vi "itc ltc plots.vi"(4 "Plot: heater/gas":refnum<vi>, 5 "aggregate every # sec":dbl=1.0, 6 "Plot: temperature":refnum<vi>, 7 "plot length (min)":dbl=20.0, 8 "plot?":bool=TRUE, 10 "temperature indicator panel":T1={"LTC T"=0.0, "ITC T"=299.2, "ITC Set T"=295.0, "LTC T slope, K/min"=-0.0, "heater i-average, V"=-0.0, "heater slope, V/min"=-0.0, "LTC T i-average, K"=0.0, "ITC T i-average, K"=0.0, "gas"=0.0} {"ITC Set T" format="%.3g"; "ITC T" format="%.3g"; "LTC T" format="%.3g"; "gas" format="%.3g"; "ITC T i-average, K" format="%#.5f"; "LTC T i-average, K" format="%#.5f"; "heater i-average, V" format="%.3g"; "heater slope, V/min" format="%#.5f"; "LTC T slope, K/min" format="%#.5f"}, 11 "time (sec)":dbl) -> ()   [LabVIEW 2015]
uses:
  temperature indicator.ctl
  aggregator - v - real - atomic.vi
  linear interpolation - real.vi
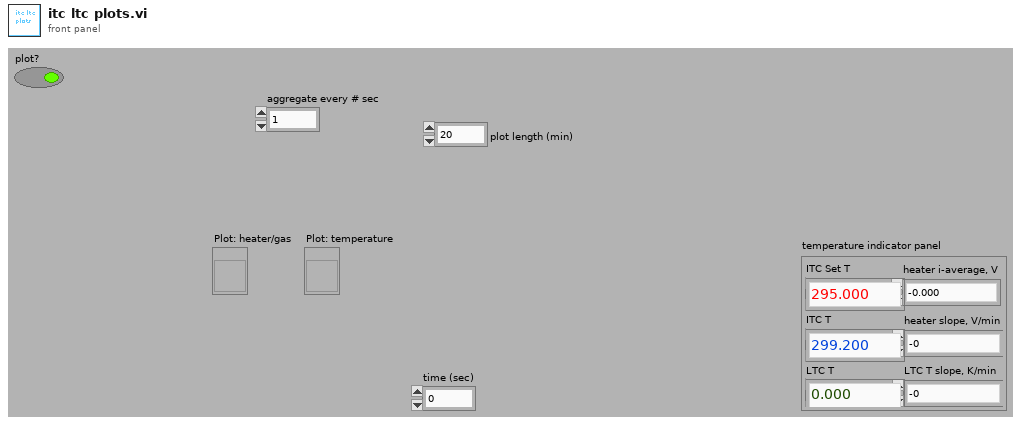
[diagram p1: front panel]
types:
  T1 = typedef "temperature indicator.ctl" = cluster{"LTC T":dbl, "ITC T":dbl, "ITC Set T":dbl, "LTC T slope, K/min":dbl, "heater i-average, V":dbl, "heater slope, V/min":dbl, "LTC T i-average, K":dbl, "ITC T i-average, K":dbl, "gas":dbl}
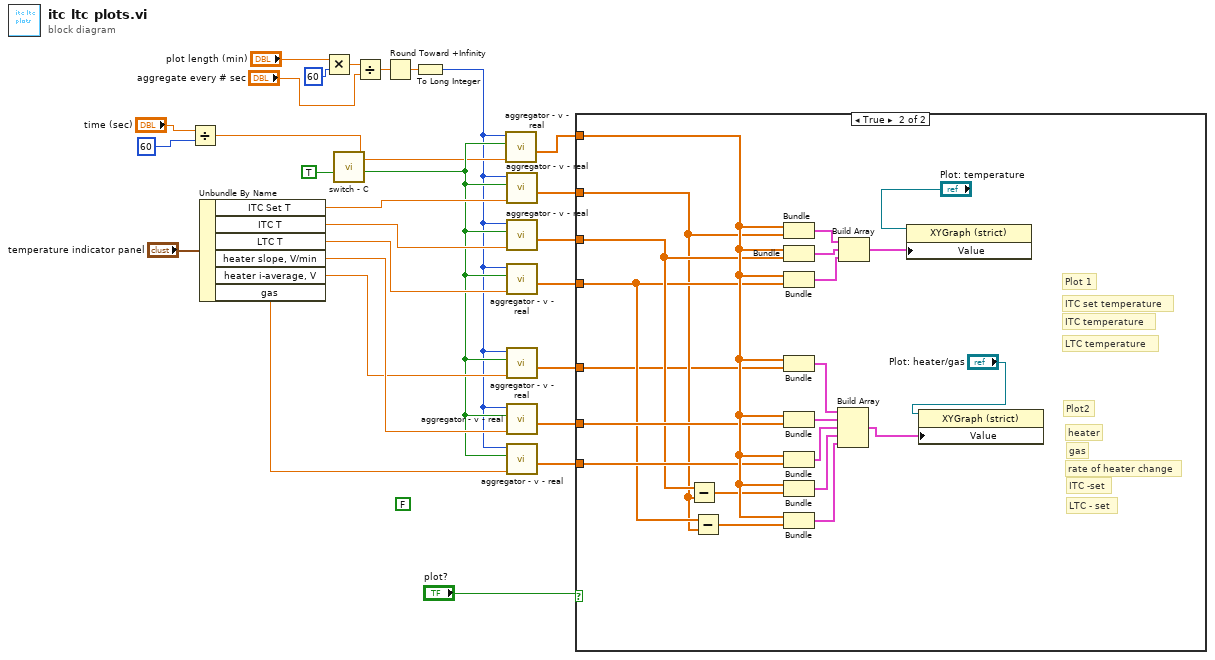
[diagram p0: block diagram]
diagram:
  (unwired) FALSE
  n1 = Divide(x="time (sec)", y=60) -> (x/y=w4:dbl)
  n2 = Unbundle By Name("temperature indicator panel") -> ("ITC Set T"=w26:dbl, "ITC T"=w25:dbl, "LTC T"=w24:dbl, "heater slope, V/min"=w15:dbl, "heater i-average, V"=w14:dbl, "gas"=w13:dbl)
  n3 = Multiply(x="plot length (min)", y=60) -> (x*y=w19:dbl)
  n4 = call "switch - C.vi"("switch"=TRUE) -> ("result"=w12:bool)  [unwired: 10 in]
  n5 = Divide(x=w19, y="aggregate every # sec") -> (x/y=w17:dbl)
  n6 = Round Toward +Infinity(x=w17) -> (ceil(x): smallest int >= x=w22:dbl)
  n7 = To Long Integer(number=w22) -> (32bit integer=w1:i32)
  n8 = call "aggregator - v - real.vi"("number"=w4, "init?"=w12, "requested size"=w1) -> ("Array"=w16:dbl[])  [unwired: 8 in]
  n9 = call "aggregator - v - real.vi"("number"=w26, "init?"=w12, "requested size"=w1) -> ("Array"=w6:dbl[])  [unwired: 8 in]
  n10 = call "aggregator - v - real.vi"("number"=w25, "init?"=w12, "requested size"=w1) -> ("Array"=w8:dbl[])  [unwired: 8 in]
  n11 = call "aggregator - v - real.vi"("number"=w24, "init?"=w12, "requested size"=w1) -> ("Array"=w7:dbl[])  [unwired: 8 in]
  n12 = call "aggregator - v - real.vi"("number"=w14, "init?"=w12, "requested size"=w1) -> ("Array"=w10:dbl[])  [unwired: 8 in]
  n13 = call "aggregator - v - real.vi"("number"=w15, "init?"=w12, "requested size"=w1) -> ("Array"=w11:dbl[])  [unwired: 8 in]
  n14 = call "aggregator - v - real.vi"("number"=w13, "init?"=w12, "requested size"=w1) -> ("Array"=w9:dbl[])  [unwired: 8 in]
  n15 = case shown="True" "plot?" {
    tunnel: w16 -> [_ w38]
    tunnel: w11 -> [_ w37]
    tunnel: w10 -> [_ w28]
    tunnel: w9 -> [_ w36]
    tunnel: w8 -> [_ w35]
    tunnel: w7 -> [_ w33]
    tunnel: w6 -> [_ w32]
    frame False {
    }
    frame True {
      # "rate of heater change"
      # "Plot2"
      # "Plot 1"
      # "ITC -set"
      # "LTC - set"
      # "gas"
      # "heater"
      # "LTC temperature"
      # "ITC temperature"
      # "ITC set temperature"
      n16 = Subtract(x=w35, y=w32) -> (x-y=w34:dbl[])
      n17 = Subtract(x=w33, y=w32) -> (x-y=w31:dbl[])
      n18 = Bundle("Array"=w38, "Array"=w32) -> (w48:cluster{"Array":dbl[], "Array":dbl[]})  [unwired: 1 in]
      n19 = Bundle("Array"=w38, "Array"=w35) -> (w42:cluster{"Array":dbl[], "Array":dbl[]})  [unwired: 1 in]
      n20 = Bundle("Array"=w38, "Array"=w33) -> (w41:cluster{"Array":dbl[], "Array":dbl[]})  [unwired: 1 in]
      n21 = Bundle("Array"=w38, "Array"=w28) -> (w43:cluster{"Array":dbl[], "Array":dbl[]})  [unwired: 1 in]
      n22 = Bundle("Array"=w38, "Array"=w37) -> (w44:cluster{"Array":dbl[], "Array":dbl[]})  [unwired: 1 in]
      n23 = Bundle("Array"=w38, "Array"=w36) -> (w45:cluster{"Array":dbl[], "Array":dbl[]})  [unwired: 1 in]
      n24 = Bundle("Array"=w38, w34) -> (w46:cluster{"Array":dbl[], dbl[]})  [unwired: 1 in]
      n25 = Bundle("Array"=w38, w31) -> (w47:cluster{"Array":dbl[], dbl[]})  [unwired: 1 in]
      n26 = Build Array(w43, w44, w45, w46, w47) -> (w29:cluster{"Array":dbl[], "Array":dbl[]}[])
      n27 = Build Array(w48, w42, w41) -> (w39:cluster{"Array":dbl[], "Array":dbl[]}[])
      n28 = property class="XYGraph (strict)"(reference="Plot: temperature", "Value"=w39) -> ()  [unwired: 1 in, 2 out]
      n29 = property class="XYGraph (strict)"(reference="Plot: heater/gas", "Value"=w29) -> ()  [unwired: 1 in, 2 out]
    }
  }
